vi "target distance and angle.vi"(10 "x side":dbl, 11 "x center":dbl) -> (2 "target angle in degrees":dbl, 3 "distance from target in inches":dbl)   [LabVIEW 2018]
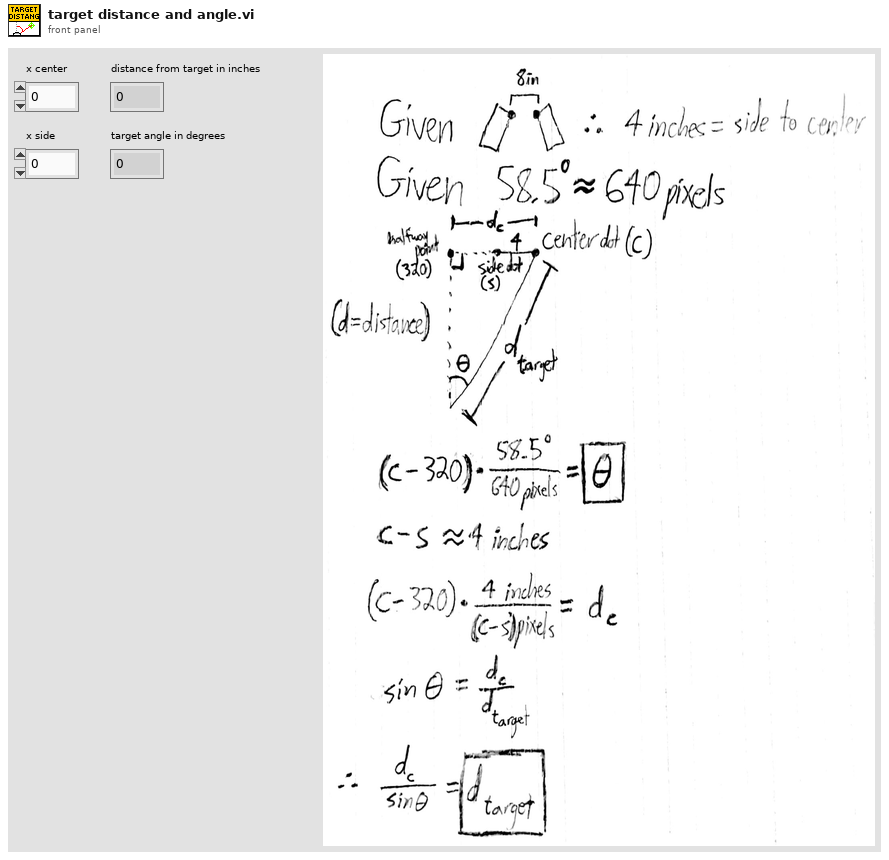
[diagram p1: front panel]
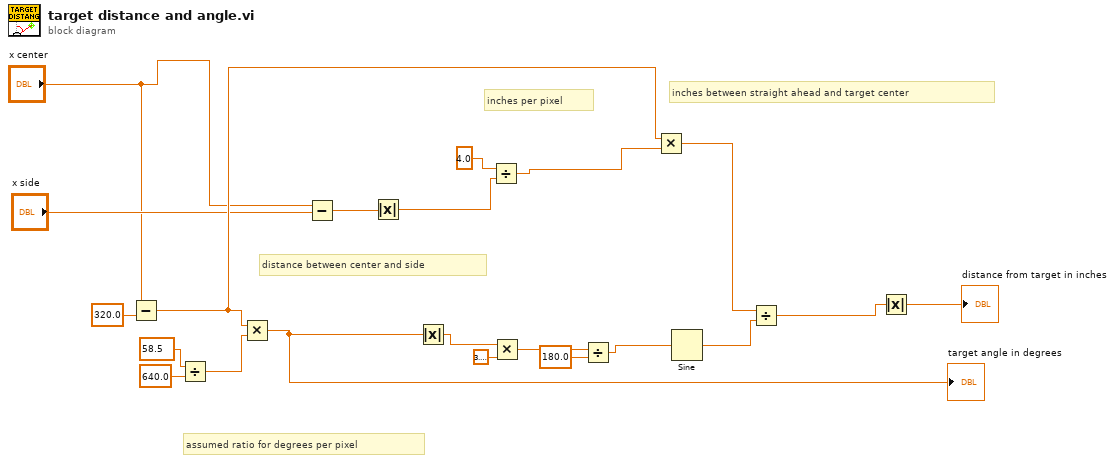
[diagram p0: block diagram]
diagram:
  # "assumed ratio for degrees per pixel"
  # "distance between center and side"
  # "inches between straight ahead and target center"
  # "inches per pixel"
  n1 = Subtract(x="x center", y=320.0) -> (x-y=w21:dbl)
  n2 = Divide(x=58.5, y=640.0) -> (x/y=w8:dbl)
  n3 = Multiply(x=w21, y=w8) -> (x*y=w9:dbl)
  "target angle in degrees" <- w9
  n4 = Subtract(x="x center", y="x side") -> (x-y=w12:dbl)
  n5 = Absolute Value(x=w12) -> (abs(x)=w13:dbl)
  n6 = Absolute Value(x=w9) -> (abs(x)=w14:dbl)
  n7 = Divide(x=4.0, y=w13) -> (x/y=w3:dbl)
  n8 = Multiply(x=w14, y=3.141592653589793) -> (x*y=w17:dbl)
  n9 = Divide(x=w17, y=180.0) -> (x/y=w18:dbl)
  n10 = Multiply(x=w21, y=w3) -> (x*y=w5:dbl)
  n11 = Sine(x=w18) -> (sin(x)=w15:dbl)
  n12 = Divide(x=w5, y=w15) -> (x/y=w16:dbl)
  n13 = Absolute Value(x=w16) -> (abs(x)=→"distance from target in inches":dbl)
